vi "folderizer_2.vi"() -> ()   [LabVIEW 2012]
panel:
  out "error out":errorcluster
  out "Copying progress (%)":dbl(slide) scale=0.0..100.0
  in  "Destination folder":path
  in  "Source folder":path
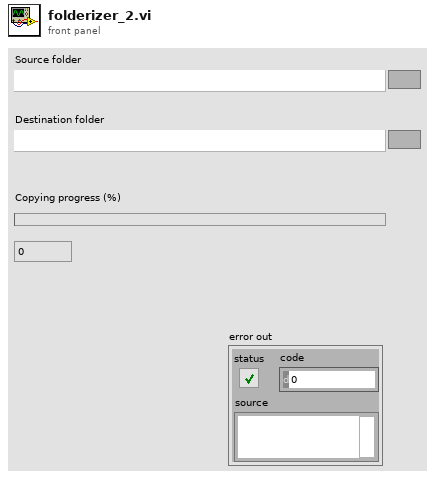
[diagram p1: front panel]
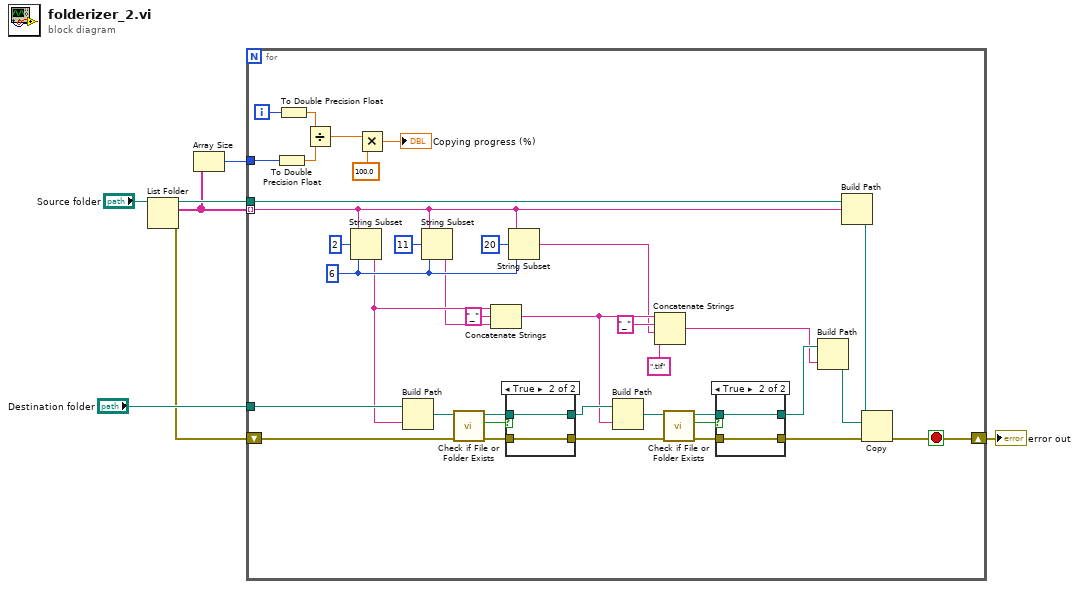
[diagram p0: block diagram]
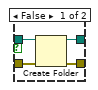
[diagram p2: hidden frame]
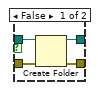
[diagram p3: hidden frame]
diagram:
  n1 = List Folder(path="Source folder") -> (path out=w6:path, filenames=w3:string[], error out=w4:errorcluster)  [unwired: 3 in, 1 out]
  n2 = Array Size(array=w3) -> (size(s)=w2:i32)
  n3 = for {
    tunnel: w3 -> [w30] mode=indexing
    tunnel: w6 -> [w31]
    tunnel: "Destination folder" -> [w45]
    shift-right: [w27] -> w1
    shift-left: w4 -> [w43]
    tunnel: w2 -> [w25]
    i -> [w26]
    stop <- w27 stop-if-true
    w19 = 6 ("length (rest)")
    n4 = To Double Precision Float(number=w25) -> (double precision float=w24:dbl)
    n5 = To Double Precision Float(number=w26) -> (double precision float=w23:dbl)
    n6 = Divide(x=w23, y=w24) -> (x/y=w22:dbl)
    n7 = String Subset(string=w30, offset (0)=2, length (rest)=w19) -> (substring=w15:string)
    n8 = Multiply(x=w22, y=100.0) -> (x*y=→"Copying progress (%)":dbl)
    n9 = Build Path(base path=w45, name or relative path=w15) -> (appended path=w44:path)
    n10 = String Subset(string=w30, offset (0)=11, length (rest)=w19) -> (substring=w14:string)
    n11 = call <vilib>:"Check if File or Folder Exists.vi"("error in (no error)"=w43, "path"=w44) -> ("error out"=w41:errorcluster, "file or folder exists?"=w42:bool, "dup path"=w40:path)  [unwired: 7 in]
    n12 = Concatenate Strings(w15, "_" ("string"), w14) -> (w11:string)
    n13 = case shown="True" w42 {
      tunnel: w41 -> [w55 w56]
      tunnel: w40 -> [w54 w57]
      tunnel: [w53 w56] -> w35
      tunnel: [w52 w57] -> w34
      frame False {
        n14 = Create Folder(path (use dialog)=w54, error in=w55) -> (created path=w52:path, error out=w53:errorcluster)  [unwired: 1 in, 1 out]
      }
      frame True {
      }
    }
    n15 = String Subset(string=w30, offset (0)=20, length (rest)=w19) -> (substring=w10:string)
    n16 = Build Path(base path=w34, name or relative path=w11) -> (appended path=w39:path)
    n17 = Concatenate Strings(w11, "_" ("string"), w10, ".tif" ("string")) -> (w8:string)
    n18 = call <vilib>:"Check if File or Folder Exists.vi"("error in (no error)"=w35, "path"=w39) -> ("error out"=w37:errorcluster, "file or folder exists?"=w38:bool, "dup path"=w36:path)  [unwired: 7 in]
    n19 = case shown="True" w38 {
      tunnel: w37 -> [w49 w50]
      tunnel: w36 -> [w48 w51]
      tunnel: [w47 w50] -> w32
      tunnel: [w46 w51] -> w33
      frame False {
        n20 = Create Folder(path (use dialog)=w48, error in=w49) -> (created path=w46:path, error out=w47:errorcluster)  [unwired: 1 in, 1 out]
      }
      frame True {
      }
    }
    n21 = Build Path(base path=w33, name or relative path=w8) -> (appended path=w28:path)
    n22 = Build Path(base path=w31, name or relative path=w30) -> (appended path=w29:path)
    n23 = Copy(8:w32, 10:w28, 11:w29) -> (0:w27:errorcluster)  [unwired: 2 in, 2 out]
  }
  "error out" <- w1
